vi "Open.vi"(8 "Error In":errorcluster, 11 "Keithley 2602 In":refnum<visa-resource-name>="GPIB0::28::INSTR") -> (0 "Error Out":errorcluster, 3 "Keithley 2602 Out":refnum<visa-resource-name>)   [LabVIEW 2012, in "Keithley-2602.lvlib"]
uses:
  Keithley-2602.lvlib
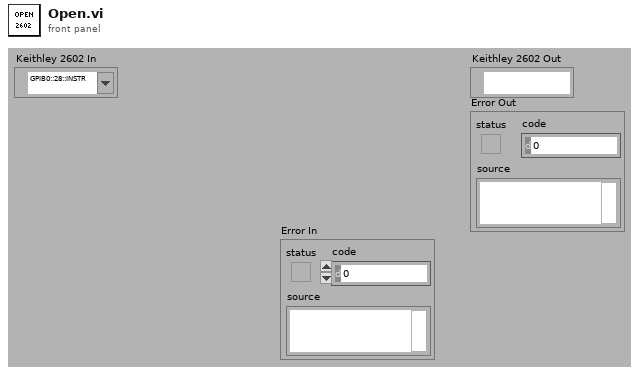
[diagram p1: front panel]
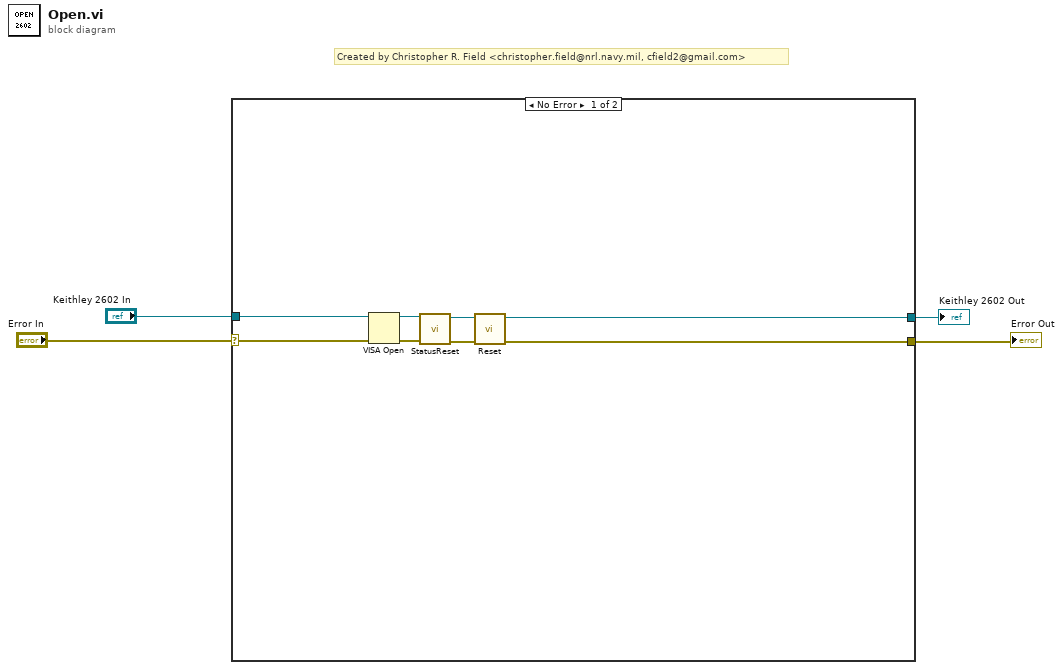
[diagram p0: block diagram]
diagram:
  # "Created by Christopher R. Field <christopher.field@nrl.navy.mil, cfield2@gmail.com>"
  n1 = case shown="No Error" "Error In" {
    selector: "Error In" -> [w5 w13]
    tunnel: "Keithley 2602 In" -> [w12 w14]
    tunnel: [w11 w14] -> w3
    tunnel: [w10 w13] -> w2
    frame No Error {
      n2 = VISA Open(error in (no error)=w5, VISA resource name=w12) -> (VISA resource name=w9:refnum<visa-resource-name>, error out=w8:errorcluster)  [unwired: 3 in]
      n3 = call "StatusReset.vi"("Error In"=w8, "Keithley 2602 In"=w9) -> ("Error Out"=w6:errorcluster, "Keithley 2602 Out"=w7:refnum<visa-resource-name>)  [unwired: 8 in]
      n4 = call "Reset.vi"("Error In"=w6, "Keithley 2602 In"=w7) -> ("Error Out"=w10:errorcluster, "Keithley 2602 Out"=w11:refnum<visa-resource-name>)  [unwired: 8 in]
    }
    frame Error {
    }
  }
  "Keithley 2602 Out" <- w3
  "Error Out" <- w2
